vi "Get Favorite Color.vi"(8 "error in":errorcluster, 11 "Team Member in":refnum<class "Team Member.lvclass">) -> (0 "error out":errorcluster, 2 "Favorite Color":u32(colorbox), 3 "Team Member out":refnum<class "Team Member.lvclass">)   [LabVIEW 2024, in "Team Member.lvclass"]
uses:
  Team Member.lvclass
  Team Member.lvclass/Team Member.ctl
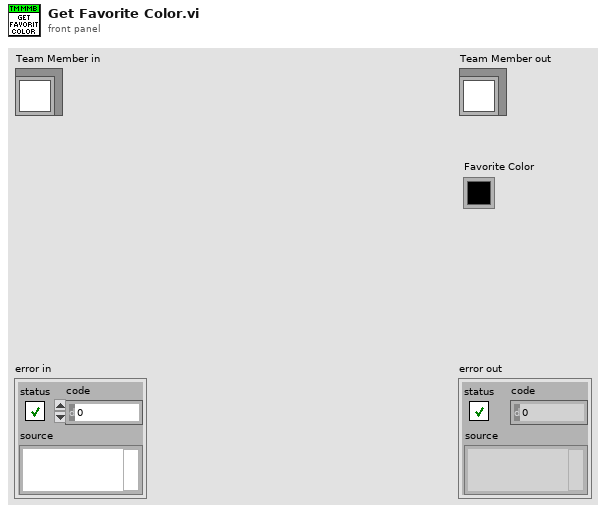
[diagram p1: front panel]
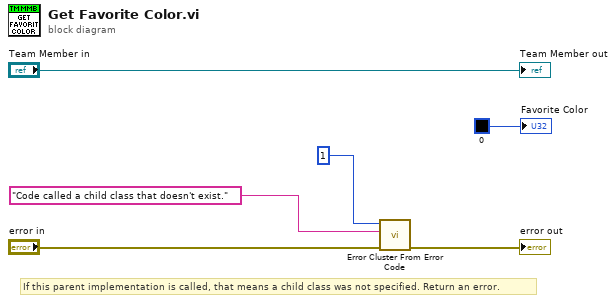
[diagram p0: block diagram]
diagram:
  # "If this parent implementation is called, that means a child class was not specified. Return an error."
  n1 = call <vilib>:"Error Cluster From Error Code.vi"("error in (no error)"="error in", "error message (\"\")"="Code called a child class that doesn't exist." ("error message (\"\")"), "error code (0)"=1) -> ("error out"=→"error out":errorcluster)  [unwired: 6 in]
  "Team Member out" <- "Team Member in"
  "Favorite Color" <- u32 0 ("Favorite Color")
